vi "Curtin1.vi"() -> ()   [LabVIEW 2022 SP3]
uses:
  ViolinSubs/Curtin1_Label.ctl
  ViolinSubs/Mic/Mic_Global.vi
  ViolinSubs/GraphType.ctl
  ViolinSubs/Perspective/subs/Perspective_Globals.vi
  <vilib>/Utility/miscctls.llb/LVPoint32TypeDef.ctl
  <vilib>/Platform/browser.llb/Open URL in Default Browser (string).vi
panel:
  in  "microphone":bool
  in  "Device":u16(ring) items=["BuerginBase Microphone", "Onyx Producer 2-2", "MacBook Pro Microphone", "Camo Microphone", "KM Audio Device", "Microsoft Teams Audio", "ZoomAudioDevice"]
  out "comma?":bool
  out "startX":i32
  out "Ctrl":bool
  out "beta":string
  in  "Settings":u16(ring) items=["Settings...", "Preferences", "Templates", "Calibrations", "Live View", "Motor Cntrl"]
  in  "ScratchPads":u16(ring) items=["Scratch...", "accelerometer taptone Scratchpad", "Admittance Scratchpad", "Laser Admitance ScratchPad", "Radiation ScratchPad", "ScratchPad", "TapTones ScratchPad"]
  in  "New Test":u16(ring) items=["New Test...", "Admittance H", "Current Settings", "Internal mic H", "JC Admit H laser", "JC Admit.HV laser", "JC H 12 radiation", "JC H 7 radiation", "JC HV 24 radiation", "Radiation H 1", "Tap repeatabilty H20"]
  in  "Help":bool
  in  "About":bool
  in  "Start":bool
  in  "email":bool
  in  "Interpret":bool
  in  "Force YRescale":bool
  out "Complex Out":cluster{dbl, "df":dbl, cdb[]}[](array[cluster])
  out "# selected":i32
  in  "Fun":bool
  out "Version":string
  in  "Preferences":bool
  in  "Set Colors":bool
  in  "Colors":u16(ring) items=["Name Current...", "Last Saved", "24 Colors", "All black", "fered", "fred", "JC"]
  in  "Share":bool
  in  "Undo":bool
  in  "Clear All":bool
  in  "select all":bool
  in  "deselect":bool
  in  "Clear":bool
  in  "Lists":bool
  in  "Browse":bool
  in  "Search":bool
  in  "Redo":bool
  in  "Files":T1[](array[typedef])
  in  "zoom":bool
  in  "Mouse Down?":bool
  in  "Views":T3={"View Type"=0, "Smoothing"=0, "Bands"=0, "Edit"=FALSE, "rescale Y"=FALSE, "rescale X"=FALSE, "X_Low"=0.0, "X_High"=0.0, "dB Range"=40.0, "Excel"=FALSE, "Y Scaling"=TRUE, "X Scaling"=TRUE, "Plot"=0} {"Plot" items=["FRF", "rad phase unwrapped", "deg phase unwrapped", "rad phase wrapped", "deg phase wrapped", "White Plots", "MJ Map", "Real and Imaginary"]; "Bands" items=["No Bands", "1 Curtin 4 (200-780-1740-2930-7000)", "1 Curtin 4a (200-780-1740-2930-6000)", "1 Curtin 5  (200-780-1740-2930-7000-10000)", "1 Curtin 5b  (200-780-1740-2930-7000-20000)", "1 Curtin 5c (250-350-780-1740-2930-7000)", "1 Curtin 5c ()", "2 Curtin (200-7000)", "3 Curtin 10 (200-340-490-640-780-1150-1390-1730-2370-2930-7000)", "4 Curtin (200-780-7000)", "Bark  (200-300-400-510-630-770-920-1080-1270-1480-1720-2000-2320-2700-3150-3700-4400-5300-6400-7700-9500)", "Curtin 4a (250-780-1740-2930-7000)", "Dunnwald (190-650-1300-1640-2580-4200-6400)", "Dunnwald (190-650-1300-4200-6400)", "Gabriellson (200-650-1080-1270-2000-3000-3700-7000)", "ivci18 rad. efficiency (200-321-618-1841-2095-3484-7790)", "Meinel (280-650-2000-3000-7000)", "ObieAlto (200-650-1575-2450-6300)", "rad. efficiency ivci (200-345-730-1192-1875-2363-3033-4040-5673)"]; "Smoothing" items=["No smoothing"=0, "1/4 semitone"=25, "1/2 semitone"=50, "1 semitone"=100, "2 semitones"=200, "3 semitones"=300, "4 semitones"=400, "Octave"=1200, "Woodhouse"=19]; "View Type" items=["As measured"=0, "Normalize"=1, "Cplx Average"=3, "Real Average"=4, "Standard Deviation"=5]}
  out "Position":string
  in  "Color Table":T4(ring)=enum."Greyscale"
  out "MJPlot":dbl[][](graph)
  out "Coords":T5
  out "White Plots":picture
  out "FRF":cluster{"x0":dbl, "df":dbl, dbl[]}[](graph)
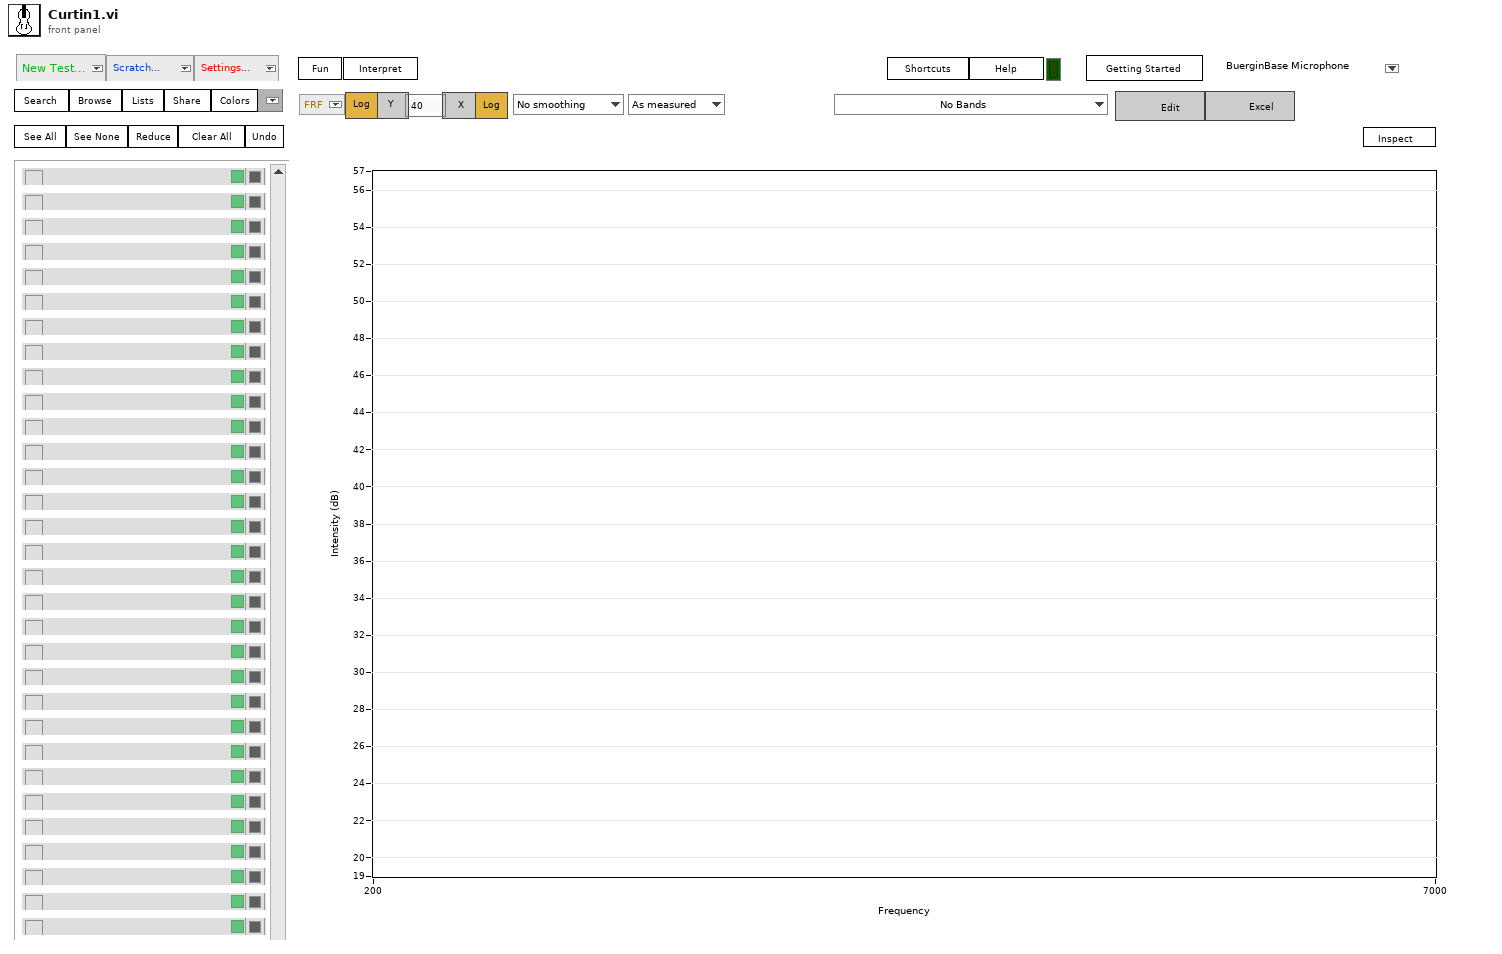
[diagram p1: front panel]
types:
  T1 = typedef "Curtin1_Label.ctl" = cluster{"Show?":bool, "Name":string, "Color":u32, "Path":path, "Show Notes":bool, "correlate":bool}
  T2 = typedef "GraphType.ctl" = u16
  T3 = cluster{"View Type":u16, "Smoothing":u16, "Bands":u16, "Edit":bool, "rescale Y":bool, "rescale X":bool, "X_Low":dbl, "X_High":dbl, "dB Range":dbl, "Excel":bool, "Y Scaling":bool, "X Scaling":bool, "Plot":T2}
  T4 = enum16{"Apricot", "Carnation", "Ether", "Greyscale", "Greyscale-banded", "Hot Metal", "Lava Waves", "Mac", "Morning Glory", "Rainbow", "Rainbow-banded", "Rainbow-inverted", "Rainbow-striped", "Saturn", "Seismic", "Space"}
  T5 = typedef "LVPoint32TypeDef.ctl" = cluster{"Horizontal":i32, "Vertical":i32}
  T6 = enum32{"SPL", "Voltage", "Accelerometer", "Vibrometer", "home", "Units"}
  T7 = enum16{"big-endian, network order", "native, host order", "little-endian"}
  T8 = enum16{"Grab Lines", "Grab Bands", "Grab Centroids"}
  T9 = cluster{"Alerts":bool, "Log X Axis":bool, "dB scale":bool, "Averaging":bool, "Fade":dbl, "Centroids?":bool, "line thickness":u8}
  T10 = typedef "LVBoundsTypeDef.ctl" = cluster{"Width":u32, "Height":u32}
  T11 = typedef "LVPositionTypeDef.ctl" = cluster{"Left":i32, "Top":i32}
  T12 = typedef "PreferencesControl.ctl" = cluster{"Name of test":string, "Date":timestamp, "Location":string, "Template":string, "Soundcard":string, "resolution":u16, "Sampling rate":u16, "Ch1 Gain ":dbl, "Ch2 Gain":dbl, "Sample time (s)":dbl, "Pre-trigger (s)":dbl, "Hammer Threshold":dbl, "Positions":i16, "Taps/Position":i16, "Set Names":string, "Freq resolution":dbl, "Hammer cutoff":dbl, "Mic cutoff":dbl, "Double bounce ":dbl, "Hammer Cal":dbl, "dB Offset":dbl, "Accel Cal":dbl, "Vibrometer Cal":dbl, "Mic Cal":dbl, "Output":u16, "Voltage Cal":dbl, "Vibrometer Port":refnum<visa-resource-name>, "Range":u16, "High Pass":u16, "Bandwidth":u16, "X Range":cluster{"Minimum":dbl, "Maximum":dbl, "Increment":dbl, "Minor Increment":dbl, "Start":dbl}[], "Y Range":cluster{"Minimum":dbl, "Maximum":dbl, "Increment":dbl, "Minor Increment":dbl, "Start":dbl}[], "dB Spread":dbl, "Trigger":u16, "Ch_1":u8, "Ch_2":u8, "flip?":bool, "60Hz":bool, "Time offset":dbl, "Piezo Cal":dbl, "Default Notes":string, "Tom":bool}
  T13 = typedef "eventvkey.ctl" = enum16{"ASCII", "Enter", "Return", "Shift", "Ctrl", "Alt", "Cmd", "Opt", "Caps", "NumLock", "Clear", "Break", "Up", "Down", "Left", "Right", "Insert", "Delete", "Home", "End", "PageUp", "PageDown", "Escape", "Help", "Pause", "ScrollLock", "F1", "F2", "F3", "F4", "F5", "F6", "F7", "F8", "F9", "F10", "F11", "F12", "F13", "F14", "F15", "F16", "F17", "F18", "F19", "F20", "F21", "F22", "F23", "F24", "Play", "VolumeUp", "VolumeDown", "Mute", "Two Byte Char"}
  T14 = typedef "LVMouseTypeDef.ctl" = cluster{"Mouse Position":cluster{"X":i32, "Y":i32}, "Mouse Modifiers":cluster{"Button Down":bool, "Shift Mod":bool, "Menu Mod":bool, "Option Mod":bool}}
  T15 = enum32{"Invalid", "Standard", "Closed", "Hidden", "Minimized", "Maximized"}
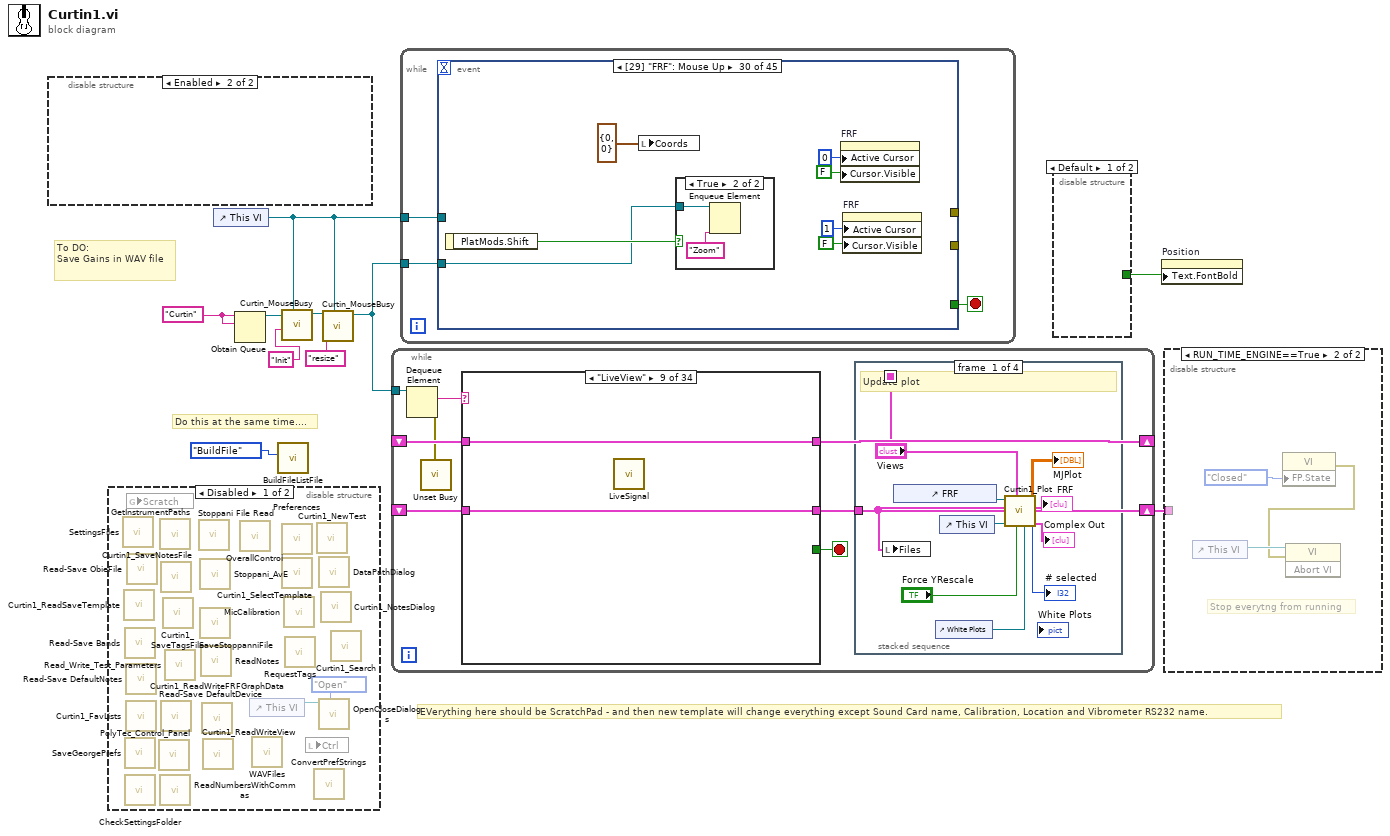
[diagram p0: block diagram]
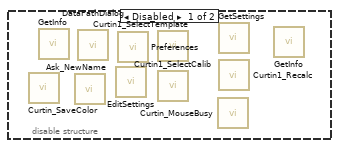
[diagram p2: hidden frame]
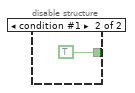
[diagram p4: hidden frame]
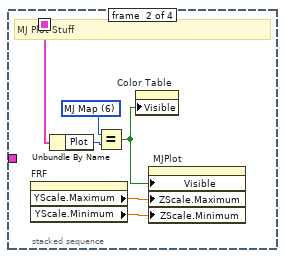
[diagram p6: hidden frame]
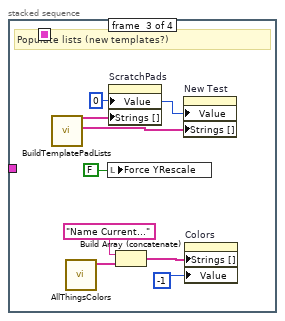
[diagram p7: hidden frame]
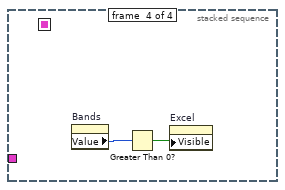
[diagram p8: hidden frame]
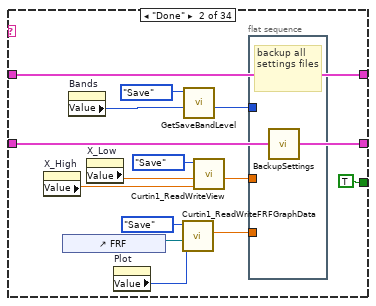
[diagram p10: hidden frame]
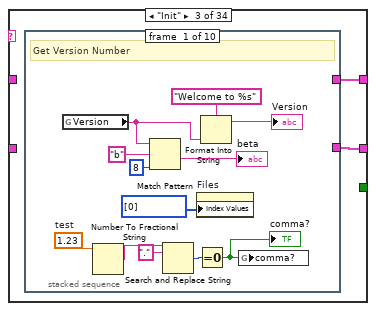
[diagram p11: hidden frame]
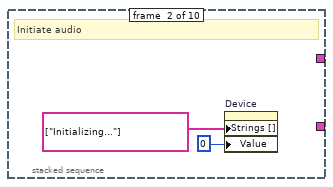
[diagram p12: hidden frame]
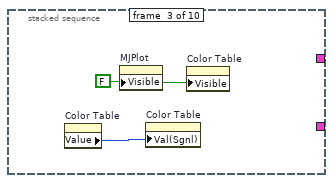
[diagram p13: hidden frame]
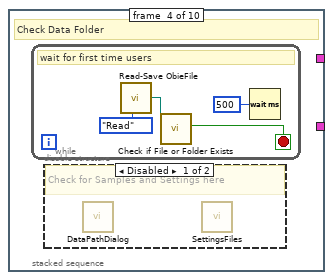
[diagram p14: hidden frame]
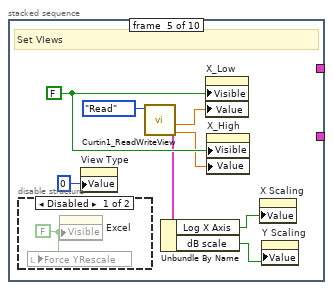
[diagram p16: hidden frame]
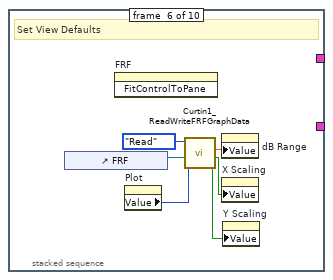
[diagram p18: hidden frame]
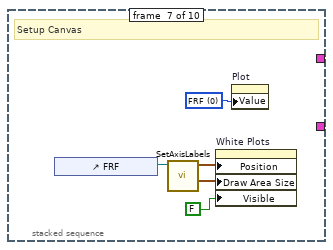
[diagram p19: hidden frame]
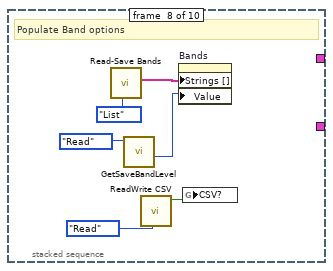
[diagram p20: hidden frame]
diagram:
  w8 = "Curtin" ("name (unnamed)")
  # "Do this at the same time...."
  # "To DO:\nSave Gains in WAV file"
  # "EVerything here should be ScratchPad - and then new template will change everything except Sound Card name, Calibration, Location and Vibrometer RS232 name."
  n1 = disable-structure shown="Enabled" {
    frame Disabled {
      n2 = call "Curtin_SaveColor.vi"() -> ()  [unwired: 10 in, 2 out]
      n3 = call "GetInfo.vi"() -> ()  [unwired: 11 in, 1 out]
      n4 = call "Ask_NewName.vi"() -> ()  [unwired: 10 in, 2 out]
      n5 = call "DataPathDialog.vi"() -> ()  [unwired: 10 in, 2 out]
      n6 = call "EditSettings.vi"() -> ()  [unwired: 10 in, 2 out]
      n7 = call "Preferences.vi"() -> ()  [unwired: 9 in, 3 out]
      n8 = call "Curtin1_SelectTemplate.vi"() -> ()  [unwired: 10 in, 2 out]
      n9 = call "Curtin1_SelectCalib.vi"() -> ()  [unwired: 11 in, 1 out]
      n10 = call "Curtin_MouseBusy.vi"() -> ()  [unwired: 11 in, 1 out]
      n11 = call "GetSettings.vi"() -> ()  [unwired: 10 in, 2 out]
      n12 = call "Curtin1_Recalc.vi"() -> ()  [unwired: 12 in]
      n13 = call "GetInfo.vi"() -> ()  [unwired: 11 in, 1 out]
    }
    frame Enabled {
    }
  }
  n14 = disable-structure shown="Disabled" {
    frame Disabled {
      n15 = call "SettingsFiles.vi"() -> ()  [unwired: 10 in, 2 out]
      n16 = call "Curtin1_ReadSaveTemplate.vi"() -> ()  [unwired: 8 in, 4 out]
      n17 = call "Read-Save Bands.vi"() -> ()  [unwired: 8 in, 4 out]
      n18 = call "SaveGeorgePrefs.vi"() -> ()  [unwired: 10 in, 2 out]
      n19 = call "CheckSettingsFolder.vi"() -> ()  [unwired: 12 in]
      n20 = call "Read-Save DefaultNotes.vi"() -> ()  [unwired: 10 in, 2 out]
      n21 = call "Curtin1_FavLists.vi"() -> ()  [unwired: 8 in, 4 out]
      n22 = global read "Mic_Global.vi" "Scratch"() -> ()  [unwired: 1 in]
      n23 = call "Read-Save ObieFile.vi"() -> ()  [unwired: 9 in, 3 out]
      n24 = call "PolyTec_Control_Panel.vi"() -> ()  [unwired: 9 in, 3 out]
      n25 = call "GetInstrumentPaths.vi"() -> ()  [unwired: 7 in, 5 out]
      n26 = call "ReadNumbersWithCommas.vi"() -> ()  [unwired: 8 in, 4 out]
      n27 = call "Curtin1_SaveNotesFile.vi"() -> ()  [unwired: 12 in]
      n28 = call "Read-Save DefaultDevice.vi"() -> ()  [unwired: 10 in, 2 out]
      n29 = call "Curtin1_SaveTagsFile.vi"() -> ()  [unwired: 12 in]
      n30 = call "Read_Write_Test_Parameters.vi"() -> ()  [unwired: 10 in, 2 out]
      n31 = call "Stoppani File Read.vi"() -> ()  [unwired: 3 in, 4 out]
      n32 = call "Stoppani_AvE.vi"() -> ()  [unwired: 8 in, 4 out]
      n33 = call "SaveStoppanniFile.vi"() -> ()  [unwired: 11 in, 1 out]
      n34 = call "ReadNotes.vi"() -> ()  [unwired: 10 in, 2 out]
      n35 = call "Curtin1_ReadWriteFRFGraphData.vi"() -> ()  [unwired: 9 in, 3 out]
      n36 = call "Curtin1_ReadWriteView.vi"() -> ()  [unwired: 9 in, 3 out]
      n37 = call "OverallControl.vi"() -> ()  [unwired: 10 in, 2 out]
      n38 = control-ref of="This VI"() -> (w11:refnum<vi>)
      n39 = call "WAVFiles.vi"() -> ()  [unwired: 8 in, 4 out]
      n40 = call "Preferences.vi"() -> ()  [unwired: 9 in, 3 out]
      n41 = call "Curtin1_SelectTemplate.vi"() -> ()  [unwired: 10 in, 2 out]
      n42 = call "MicCalibration.vi"() -> ()  [unwired: 11 in, 1 out]
      n43 = call "RequestTags.vi"() -> ()  [unwired: 11 in, 1 out]
      n44 = local read "Ctrl"() -> ()  [unwired: 1 in]
      n45 = call "ConvertPrefStrings.vi"() -> ()  [unwired: 10 in, 2 out]
      n46 = call "Curtin1_NewTest.vi"() -> ()  [unwired: 10 in, 2 out]
      n47 = call "DataPathDialog.vi"() -> ()  [unwired: 10 in, 2 out]
      n48 = call "OpenCloseDialogs.vi"("Task"=enum16{"Open", "Close"}."Open", "VI in"=w11) -> ()  [unwired: 8 in, 2 out]
      n49 = call "Curtin1_NotesDialog.vi"() -> ()  [unwired: 9 in, 3 out]
      n50 = call "Curtin1_Search.vi"() -> ()  [unwired: 10 in, 2 out]
    }
    frame Enabled {
    }
  }
  n51 = control-ref of="This VI"() -> (w3:refnum<vi>)
  n52 = Obtain Queue(name (unnamed)=w8, element data type=w8) -> (queue out=w7:refnum<queue>)  [unwired: 3 in, 2 out]
  n53 = call "BuildFileListFile.vi"("Task"=enum16{"BuildFile", "ReadFile"}."BuildFile") -> ()  [unwired: 9 in, 2 out]
  n54 = call "Curtin_MouseBusy.vi"("VI in"=w3, "element"="Init", "queue in"=w7) -> ("queue out"=w5:refnum<queue>)  [unwired: 8 in]
  n55 = call "Curtin_MouseBusy.vi"("VI in"=w3, "element"="resize", "queue in"=w5) -> ("queue out"=w6:refnum<queue>)  [unwired: 8 in]
  n56 = while {
    tunnel: w6 -> [w19]
    shift-right: [w16] -> w9
    shift-left: _ -> [w17]
    shift-right: [w14] -> _
    shift-left: _ -> [w15]
    stop <- w18 stop-if-true
    n57 = Dequeue Element(queue=w19) -> (element=w20:string, error out=w13:errorcluster)  [unwired: 2 in, 2 out]
    n58 = call <vilib>:"Unset Busy.vi"("error in (no error)"=w13) -> ()  [unwired: 10 in, 1 out]
    n59 = case shown="\"LiveView\"" w20 {
      selector: w20 -> [_ _ _ _ _ _ _ _ _ _ _ _ _ _ _ _ _ _ _ _ _ _ _ _ _ _ _ _ _ _ w301 w304 _ _]
      tunnel: [_ TRUE ("Discard?") _ _ _ _ _ _ _ _ _ _ _ _ _ _ _ _ _ _ _ _ _ _ _ _ _ _ _ _ _ _ _ _] -> w18
      tunnel: w17 -> [w48 w61 _ _ w129 w138 w154 w159 w161 w163 w165 w178 w185 w190 w201 w210 w222 w226 w228 w230 w234 w239 w242 w245 w258 w270 w276 w281 w286 w291 w302 w305 w312 w335]
      tunnel: [w48 w61 w63 w117 w129 w140 w154 w159 w161 w163 w169 w177 w186 w192 w196 w210 w221 w226 w228 w230 w232 w238 w241 w245 w257 w269 w275 w283 T1[] [] ("Files") w293 w302 w305 w312 w335] -> w16
      tunnel: [w47 w60 w64 w118 w132 w142 w155 w160 w162 w164 w167 w179 w187 w193 w202 w211 w224 w227 w229 w231 w235 w240 w243 w246 w259 w268 w274 w280 w287 w294 w303 w306 w316 w336] -> w14
      tunnel: w15 -> [w47 w60 _ w119 w132 w142 w155 w160 w162 w164 w168 w180 w188 w194 w203 w211 w225 w227 w229 w231 w236 w240 w243 w246 w260 w268 w274 w282 w289 w292 w303 w306 w316 w336]
      frame Default {
      }
      frame "Done" {
        n60 = property on="X_High" class="DigNum (strict)"() -> ("Value"=w55:dbl)  [unwired: 2 in, 2 out]
        n61 = control-ref of="FRF"() -> (w58:refnum<vi>)
        n62 = property on="Bands" class="Ring (strict)"() -> ("Value"=w53:u16)  [unwired: 2 in, 2 out]
        n63 = property on="X_Low" class="DigNum (strict)"() -> ("Value"=w56:dbl)  [unwired: 2 in, 2 out]
        n64 = property on="Plot" class="Ring (strict)"() -> ("Value"=w49:T2)  [unwired: 2 in, 2 out]
        n65 = call "Curtin1_ReadWriteFRFGraphData.vi"("Type"=w49, "FRF"=w58, "Task"=enum16{"Read", "Save"}."Save") -> ("dB"=w50:dbl)  [unwired: 6 in, 2 out]
        n66 = call "GetSaveBandLevel.vi"("Value in"=w53, "Task"=enum16{"Read", "Save"}."Save") -> ("Value out"=w52:u16)  [unwired: 9 in]
        n67 = call "Curtin1_ReadWriteView.vi"("X_High"=w55, "X_Low"=w56, "Task"=enum16{"Read", "Save"}."Save") -> ("X_Low out"=w51:dbl)  [unwired: 6 in, 2 out]
        n68 = flat-sequence {
          tunnel: w52 -> [_]
          tunnel: w51 -> [_]
          tunnel: w50 -> [_]
          frame #0 {
            # "backup all settings files"
            n69 = call "BackupSettings.vi"() -> ()  [unwired: 12 in]
          }
        }
      }
      frame "Init" {
        n70 = stacked-sequence {
          tunnel: [_ _ _ _ _ _ _ _ _ cluster{"files":T1[]}[] [] ("Array in")] -> w64
          tunnel: [_ _ _ _ _ _ _ _ _ T1[] [] ("Files")] -> w63
          frame #0 {
            w66 = 1.23  # test
            # "Get Version Number"
            n71 = global read "Mic_Global.vi" "Version"() -> (w70:string)
            n72 = Number To Fractional String(number=w66) -> (F-format string=w65:string)  [unwired: 3 in]
            n73 = Match Pattern(string=w70, regular expression="b", offset (0)=8) -> (after substring=→"beta":string)  [unwired: 3 out]
            n74 = Search and Replace String(input string=w65, search string=".") -> (number of replacements=w69:i32)  [unwired: 6 in, 3 out]
            n75 = property on="Files" class="Arr"("Index Values"=u32[] [0]) -> ()  [unwired: 2 in, 2 out]
            n76 = Equal To 0?(x=w69) -> (x = 0?=w67:bool)
            "comma?" <- w67
            n77 = Format Into String(format string="Welcome to %s", w70) -> (resulting string=→"Version":string)  [unwired: 2 in, 1 out]
            n78 = global write "Mic_Global.vi" "comma?"(w67) -> ()
          }
          frame #1 {
            # "Initiate audio"
            n79 = property on="Device" class="Ring (strict)"("Strings []"=string[] ["Initializing..."] ("Strings [4]"), "Value"=0) -> ()  [unwired: 2 in, 2 out]
          }
          frame #2 {
            w80 = FALSE ("Visible")
            n80 = property on="Color Table" class="Enum (strict)"() -> ("Value"=w79:T4)  [unwired: 2 in, 2 out]
            n81 = property on="MJPlot" class="IntGraph (strict)"("Visible"=w80) -> ()  [unwired: 2 in, 2 out]
            n82 = property on="Color Table" class="Enum (strict)"("Val(Sgnl)"=w79) -> ()  [unwired: 2 in, 2 out]
            n83 = property on="Color Table" class="Enum (strict)"("Visible"=w80) -> ()  [unwired: 2 in, 2 out]
          }
          frame #3 {
            # "Check Data Folder"
            n84 = while {
              stop <- w82 stop-if-true
              # "wait for first time users"
              n85 = call "Read-Save ObieFile.vi"("Task"=enum16{"Save", "Read"}."Read") -> ("DataPath Out"=w84:path)  [unwired: 8 in, 2 out]
              n86 = call <vilib>:"Check if File or Folder Exists.vi"("path"=w84) -> ("file or folder exists?"=w82:bool)  [unwired: 8 in, 2 out]
              n87 = Wait (ms)(milliseconds to wait=u32 500) -> ()  [unwired: 1 out]
            }
            n88 = disable-structure shown="Disabled" {
              frame Disabled {
                # "Check for Samples and Settings here"
                n89 = call "DataPathDialog.vi"() -> ()  [unwired: 10 in, 2 out]
                n90 = call "SettingsFiles.vi"() -> ()  [unwired: 10 in, 2 out]
              }
              frame Enabled {
              }
            }
          }
          frame #4 {
            w92 = FALSE ("Visible")
            # "Set VIews"
            n91 = disable-structure shown="Disabled" {
              frame Disabled {
                w93 = FALSE ("Visible")
                n92 = local write "Force YRescale"(w93) -> ()
                n93 = property on="Excel" class="Bool"("Visible"=w93) -> ()  [unwired: 2 in, 2 out]
              }
              frame Enabled {
              }
            }
            n94 = property on="View Type" class="Ring (strict)"("Value"=u16 0) -> ()  [unwired: 2 in, 2 out]
            n95 = call "Curtin1_ReadWriteView.vi"("Task"=enum16{"Read", "Save"}."Read") -> ("X_High out"=w89:dbl, "X_Low out"=w90:dbl, "View"=w85:T9)  [unwired: 8 in]
            n96 = Unbundle By Name(w85) -> ("Log X Axis"=w86:bool, "dB scale"=w87:bool)
            n97 = property on="X_Low" class="DigNum (strict)"("Visible"=w92, "Value"=w90) -> ()  [unwired: 2 in, 2 out]
            n98 = property on="X_High" class="DigNum (strict)"("Visible"=w92, "Value"=w89) -> ()  [unwired: 2 in, 2 out]
            n99 = property on="X Scaling" class="Bool (strict)"("Value"=w86) -> ()  [unwired: 2 in, 2 out]
            n100 = property on="Y Scaling" class="Bool (strict)"("Value"=w87) -> ()  [unwired: 2 in, 2 out]
          }
          frame #5 {
            # "Set View Defaults"
            n101 = control-ref of="FRF"() -> (w99:refnum<vi>)
            n102 = invoke on="FRF" class="WFGraph (strict)" method="FitControlToPane"() -> ()  [unwired: 3 in, 3 out]
            n103 = property on="Plot" class="Ring (strict)"() -> ("Value"=w96:T2)  [unwired: 2 in, 2 out]
            n104 = call "Curtin1_ReadWriteFRFGraphData.vi"("Type"=w96, "FRF"=w99, "Task"=enum16{"Read", "Save"}."Read") -> ("y log?"=w95:bool, "x log?"=w94:bool, "dB"=w97:dbl)  [unwired: 6 in]
            n105 = property on="dB Range" class="DigNum (strict)"("Value"=w97) -> ()  [unwired: 2 in, 2 out]
            n106 = property on="X Scaling" class="Bool (strict)"("Value"=w94) -> ()  [unwired: 2 in, 2 out]
            n107 = property on="Y Scaling" class="Bool (strict)"("Value"=w95) -> ()  [unwired: 2 in, 2 out]
          }
          frame #6 {
            w100 = T2 0 items=["FRF", "rad phase unwrapped", "deg phase unwrapped", "rad phase wrapped", "deg phase wrapped", "White Plots"] ("Value")
            # "Setup Canvas"
            n108 = control-ref of="FRF"() -> (w104:refnum<vi>)
            n109 = call "SetAxisLabels.vi"("WaveformGraph in"=w104) -> ("Bounds"=w102:T10, "Position"=w103:T11)  [unwired: 8 in, 1 out]
            n110 = property on="White Plots" class="Pict"("Position"=w103, "Draw Area Size"=w102, "Visible"=FALSE) -> ()  [unwired: 2 in, 2 out]
            n111 = property on="Plot" class="Ring (strict)"("Value"=w100) -> ()  [unwired: 2 in, 2 out]
          }
          frame #7 {
            # "Populate Band options"
            n112 = call "Read-Save Bands.vi"("Task"=enum16{"Save", "Read", "List"}."List") -> ("Long names"=w110:string[])  [unwired: 7 in, 3 out]
            n113 = call "GetSaveBandLevel.vi"("Task"=enum16{"Read", "Save"}."Read") -> ("Value out"=w107:u16)  [unwired: 10 in]
            n114 = call "ReadWrite CSV.vi"("Task"=enum16{"Save", "Read"}."Read") -> ("csv Out"=w105:bool)  [unwired: 10 in]
            n115 = property on="Bands" class="Ring (strict)"("Strings []"=w110, "Value"=w107) -> ()  [unwired: 2 in, 2 out]
            n116 = global write "Mic_Global.vi" "CSV?"(w105) -> ()
          }
          frame #8 {
            # "Always start everyone with ScratchPad \n\nRead the latest calibration but do not \ndo anything with it (no error code/saving)"
            # "Upload  ScratchPad template"
            n117 = call "UpdateScratchPad.vi"() -> ("Settings Out"=w112:T12)  [unwired: 10 in, 1 out]
            n118 = global write "Mic_Global.vi" "Settings"(w112) -> ()
            n119 = control-ref of="Device"() -> (w113:refnum<vi>)
            n120 = call "Curtin1_soundcards.vi"("hush?"=TRUE, "Settings In"=w112, "device:"=w113) -> ()  [unwired: 7 in, 2 out]
          }
          frame #9 {
            # "Initialize Undo and List"
          }
        }
      }
      frame "Update" {
        # "NOTE: info box is in this frame"
        n121 = call "Curtin1_NotesDialog.vi"("Files"="Files") -> ("Color"=w121:u32[], "removed?"=w120:bool, "Array"=w117:T1[])  [unwired: 8 in]
        n122 = call "Curtin1_Color.vi"("Color"=w121) -> ()  [unwired: 9 in, 2 out]
        n123 = case shown="True" w120 {
          tunnel: w119 -> [w123 w126]
          tunnel: [w123 w125] -> w118
          tunnel: w117 -> [_ w124]
          frame False {
          }
          frame True {
            # "removed a plot"
            n124 = call "Curtin_Undo.vi"("New Files"=w124, "Array in"=w126) -> ("Array out"=w125:cluster{"files":T1[]}[])  [unwired: 9 in]
          }
        }
        n125 = property on="Colors" class="Ring (strict)"("Value"=-1) -> ()  [unwired: 2 in, 2 out]
      }
      frame "Zoom" {
        n126 = for {
          tunnel: w129 -> [w135] mode=indexing
          tunnel: [w134] -> w128 mode=indexing if=w133
          n127 = Unbundle By Name(w135) -> ("Name"=w134:string, "Show?"=w133:bool)
        }
        n128 = property on="Plot" class="Ring (strict)"() -> ("Value"=w127:T2)  [unwired: 2 in, 2 out]
        n129 = property on="dB Range" class="DigNum (strict)"() -> ("Value"=w130:dbl)  [unwired: 2 in, 2 out]
        n130 = control-ref of="FRF"() -> (w131:refnum<vi>)
        n131 = call "GraphZoom.vi"("Plot"=w127, "Names"=w128, "dB Range"=w130, "Graph"=w131) -> ()  [unwired: 8 in]
      }
      frame "Preferences" {
        n132 = control-ref of="Files"() -> (w141:refnum<vi>)
        n133 = call "Preferences.vi"("FileList"=w141, "Files"=w138) -> ("Settings out"=w136:T12, "Success?"=w139:bool, "Fixed Files"=w137:T1[])  [unwired: 7 in]
        n134 = case shown="True" w139 {
          tunnel: w137 -> [_ w151]
          tunnel: [w143 w151] -> w140
          tunnel: w138 -> [w143 _]
          tunnel: w136 -> [_ w147]
          frame False {
          }
          frame True {
            n135 = global read "Mic_Global.vi" "View"() -> (w150:T9)
            n136 = call "UpdateScratchPad.vi"("Settings"=w147) -> ("Settings Out"=w144:T12)  [unwired: 9 in, 1 out]
            n137 = Unbundle By Name(w150) -> ("Log X Axis"=w149:bool, "dB scale"=w148:bool)
            n138 = control-ref of="Device"() -> (w146:refnum<vi>)
            n139 = call "Curtin1_soundcards.vi"("hush?"=TRUE, "Settings In"=w144, "device:"=w146) -> ()  [unwired: 7 in, 2 out]
            n140 = property on="X Scaling" class="Bool (strict)"("Value"=w149) -> ()  [unwired: 2 in, 2 out]
            n141 = property on="Y Scaling" class="Bool (strict)"("Value"=w148) -> ()  [unwired: 2 in, 2 out]
          }
        }
      }
      frame "Templates" {
        n142 = global read "Mic_Global.vi" "Scratch"() -> (w153:string)
        n143 = call "EditSettings.vi"("Template in"=w153) -> ("Settings out"=w152:T12)  [unwired: 9 in, 1 out]
        n144 = call "UpdateScratchPad.vi"("Settings"=w152) -> ()  [unwired: 9 in, 2 out]
      }
      frame "Calibrations" {
        # "Saves a new calib file\nand it is pushed in test"
        n145 = call "UpdateScratchPad.vi"() -> ("Settings Out"=w157:T12)  [unwired: 10 in, 1 out]
        n146 = call "MicCalibration.vi"("Type"=T6."home" ("Tyoe"), "Settings"=w157) -> ("Settings Out"=w156:T12)  [unwired: 9 in]
        n147 = global write "Mic_Global.vi" "Settings"(w156) -> ()
        n148 = call "UpdateScratchPad.vi"("Settings"=w156) -> ()  [unwired: 9 in, 2 out]
      }
      frame "LiveView" {
        n149 = call "LiveSignal.vi"() -> ()  [unwired: 12 in]
      }
      frame "MotorControl" {
        n150 = call "MotorControl.vi"() -> ()  [unwired: 12 in]
      }
      frame "Browse" {
        n151 = Array Size(array=w165) -> (size(s)=w166:i32)
        n152 = case shown="0" w166 {
          frame Default {
          }
          frame 0 {
            n153 = local write "Force YRescale"(TRUE ("Force YRescale")) -> ()
          }
        }
        n154 = call "Curtin_Undo.vi"("New Files"=w165, "Array in"=w168) -> ("Array out"=w167:cluster{"files":T1[]}[])  [unwired: 9 in]
        n155 = call "Curtin1_LoadFile.vi"("Files in"=w165) -> ("Files out"=w169:T1[])  [unwired: 10 in]
      }
      frame "Preload" {
        n156 = call "Curtin1_GlobalFolder.vi"() -> ("Samples"=w171:path)  [unwired: 1 in, 1 out]
        n157 = List Folder(path=w171, pattern="*.AvC") -> (path out=w174:path, filenames=w173:string[])  [unwired: 2 in, 2 out]
        n158 = call "Curtin_Undo.vi"("New Files"=w178, "Array in"=w180) -> ("Array out"=w179:cluster{"files":T1[]}[])  [unwired: 9 in]
        n159 = local write "Force YRescale"(TRUE ("Force YRescale")) -> ()
        n160 = for {
          tunnel: w174 -> [w183]
          tunnel: w173 -> [w182] mode=indexing
          tunnel: [w181] -> w172 mode=indexing
          n161 = Build Path(base path=w183, name or relative path=w182) -> (appended path=w181:path)
        }
        n162 = call "Curtin1_AddTest.vi"("Selected Paths"=w172) -> ("New Files"=w177:T1[])  [unwired: 10 in]
      }
      frame "Search" {
        n163 = Array Size(array=w185) -> (size(s)=w184:i32)
        n164 = case shown="0" w184 {
          frame Default {
          }
          frame 0 {
            n165 = local write "Force YRescale"(TRUE ("Force YRescale")) -> ()
          }
        }
        n166 = call "Curtin_Undo.vi"("New Files"=w185, "Array in"=w188) -> ("Array out"=w187:cluster{"files":T1[]}[])  [unwired: 9 in]
        n167 = call "Curtin1_Search.vi"("Old Files"=w185) -> ("New Files"=w186:T1[])  [unwired: 9 in, 1 out]
      }
      frame "Lists" {
        n168 = Array Size(array=w190) -> (size(s)=w191:i32)
        n169 = case shown="0" w191 {
          frame Default {
          }
          frame 0 {
            n170 = local write "Force YRescale"(TRUE ("Force YRescale")) -> ()
          }
        }
        n171 = call "Curtin_Undo.vi"("New Files"=w190, "Array in"=w194) -> ("Array out"=w193:cluster{"files":T1[]}[])  [unwired: 9 in]
        n172 = call "Curtin1_Lists.vi"("Old Files"=w190) -> ("New Files"=w192:T1[])  [unwired: 10 in]
      }
      frame "newColors" {
        n173 = property on="Colors" class="Ring (strict)"() -> ("Strings []"=w199:string[], "Value"=w200:u16)  [unwired: 2 in, 2 out]
        n174 = Index Array(array=w199, index=w200) -> (element=w198:string)
        n175 = call "AllThingsColors.vi"("Choice"=w198) -> ("Possible Colors"=w197:string[])  [unwired: 10 in]
        n176 = for {
          tunnel: w201 -> [w207] mode=indexing
          tunnel: [w206] -> w196 mode=indexing
          tunnel: w197 -> [_]
          i -> [w205]
          n177 = call "Curtin1_Color.vi"("Offset"=w205) -> ("New color"=w204:u32)  [unwired: 9 in, 1 out]
          n178 = Bundle By Name(cluster=w207, "Color"=w204) -> (w206:T1)
        }
        n179 = call "Curtin_Undo.vi"("New Files"=w201, "Array in"=w203) -> ("Array out"=w202:cluster{"files":T1[]}[])  [unwired: 9 in]
        n180 = local write "Files"(w196) -> ()
      }
      frame "saveColors" {
        n181 = call "Curtin_SaveColor.vi"() -> ("New Color"=w209:string, "Good?"=w208:bool)  [unwired: 10 in]
        n182 = case shown="True" w208 {
          tunnel: w210 -> [_ w215]
          tunnel: w209 -> [_ w213]
          tunnel: [_ w214] -> _
          frame False {
          }
          frame True {
            n183 = for {
              tunnel: w215 -> [w220] mode=indexing
              tunnel: [w219] -> w218 mode=indexing
              n184 = Unbundle By Name(w220) -> ("Color"=w219:u32)
            }
            n185 = call "GetColorFilePath.vi"("String"=w213) -> ("path"=w212:path)  [unwired: 9 in, 1 out]
            n186 = Write to Binary File(file (use dialog)=w212, data=w218, 5:FALSE ("prepend array or string size? (T)"), 9:T7."big-endian, network order" ("byte order (0:big-endian, network order)")) -> (error out=w214:errorcluster)  [unwired: 2 in, 2 out]
          }
        }
      }
      frame "setColors" {
        n187 = control-ref of="Files"() -> (w223:refnum<vi>)
        n188 = call "DefineColorPalette.vi"("Files in"=w222, "FileList"=w223) -> ("Files out"=w221:T1[])  [unwired: 9 in]
        n189 = call "Curtin_Undo.vi"("New Files"=w222, "Array in"=w225) -> ("Array out"=w224:cluster{"files":T1[]}[])  [unwired: 9 in]
      }
      frame "Fun" {
        n190 = call "FunArea.vi"("Old Files"=w226) -> ()  [unwired: 11 in]
      }
      frame "PlayIt" {
        n191 = call "PlayFile.vi"("Old Files"=w228) -> ()  [unwired: 11 in]
      }
      frame "Share" {
        n192 = call "Curtin1_Share.vi"("Files"=w230) -> ()  [unwired: 11 in]
      }
      frame "AppendTest" {
        n193 = global read "Mic_Global.vi" "Settings"() -> (w233:T12)
        n194 = call "Curtin1_DAQFiles.vi"("Settings"=w233, "Files in"=w234) -> ("Files out"=w232:T1[])  [unwired: 9 in]
        n195 = call "Curtin_Undo.vi"("New Files"=w234, "Array in"=w236) -> ("Array out"=w235:cluster{"files":T1[]}[])  [unwired: 9 in]
        n196 = flat-sequence {
          tunnel: w232 -> [_]
          frame #0 {
            n197 = call "BuildFileListFile.vi"("Task"=enum16{"BuildFile", "ReadFile"}."BuildFile") -> ()  [unwired: 9 in, 2 out]
          }
        }
      }
      frame "woodhouse" {
        n198 = call "Woodhouse.vi"("Files in"=w239) -> ("Files out"=w238:T1[])  [unwired: 10 in]
      }
      frame "SamZ" {
        n199 = call "SamZ_Format.vi"("Files in"=w242) -> ("Files out"=w241:T1[])  [unwired: 10 in]
      }
      frame "Folder" {
        n200 = for {
          tunnel: w245 -> [w251] mode=indexing
          tunnel: [w250] -> w244 mode=indexing if=w249
          n201 = Unbundle By Name(w251) -> ("Path"=w250:path, "Show?"=w249:bool)
        }
        n202 = for {
          tunnel: w244 -> [w248] mode=indexing
          n203 = Strip Path(path=w248) -> (stripped path=w247:path)  [unwired: 1 out]
          n204 = call "OpenFolder.vi"("LabVIEW Data Path"=w247) -> ()  [unwired: 11 in]
        }
      }
      frame "AppendAve" {
        n205 = local read "Complex Out"() -> (w256:cluster{dbl, "df":dbl, cdb[]}[])
        n206 = property on="View Type" class="Ring (strict)"() -> ("Value"=w254:u16)  [unwired: 2 in, 2 out]
        n207 = local read "# selected"() -> (w255:i32)
        n208 = call "SaveGroupAverages.vi"("nAverages"=w255, "Value"=w254, "Complex"=w256) -> ("New Path"=w252:path)  [unwired: 8 in]
        n209 = Not A Number/Path/Refnum?(number/path/refnum=w252) -> (NaN/Path/Refnum?=w253:bool)
        n210 = call "Curtin_Undo.vi"("New Files"=w258, "Array in"=w260) -> ("Array out"=w259:cluster{"files":T1[]}[])  [unwired: 9 in]
        n211 = case shown="False" w253 {
          tunnel: w258 -> [w265 w267]
          tunnel: [w264 w267] -> w257
          tunnel: w252 -> [w263 _]
          frame False {
            n212 = Build Array(w263) -> (w262:path[])
            n213 = call "Curtin1_AddTest.vi"("Old Files"=w265, "Selected Paths"=w262) -> ("New Files"=w264:T1[])  [unwired: 9 in]
            n214 = property on="View Type" class="Ring (strict)"("Val(Sgnl)"=0) -> ()  [unwired: 2 in, 2 out]
            n215 = call "BuildFileListFile.vi"("Task"=enum16{"BuildFile", "ReadFile"}."BuildFile") -> ()  [unwired: 9 in, 2 out]
          }
          frame True {
          }
        }
      }
      frame "Deselect" {
        n216 = for {
          tunnel: w270 -> [w273] mode=indexing
          tunnel: [w272] -> w269 mode=indexing
          n217 = Bundle By Name(cluster=w273, "Show?"=FALSE) -> (w272:T1)
        }
      }
      frame "SelectAll" {
        n218 = for {
          tunnel: w276 -> [w279] mode=indexing
          tunnel: [w278] -> w275 mode=indexing
          n219 = Bundle By Name(cluster=w279, "Show?"=TRUE) -> (w278:T1)
        }
      }
      frame "Clear" {
        n220 = call "Curtin_Undo.vi"("New Files"=w281, "Array in"=w282) -> ("Array out"=w280:cluster{"files":T1[]}[])  [unwired: 9 in]
        n221 = for {
          tunnel: w281 -> [w285] mode=indexing
          tunnel: [w285] -> w283 mode=indexing if=w284
          n222 = Unbundle By Name(w285) -> ("Show?"=w284:bool)
        }
      }
      frame "Clear All" {
        n223 = call "Curtin_Undo.vi"("New Files"=w286, "Array in"=w289) -> ("Array out"=w287:cluster{"files":T1[]}[])  [unwired: 9 in]
      }
      frame "Undo" {
        n224 = Array Size(array=w292) -> (size(s)=w290:i32)
        n225 = case shown="Default" w290 {
          tunnel: [w296 w300] -> w294
          tunnel: [w295 w297] -> w293
          tunnel: w292 -> [w296 w298]
          tunnel: w291 -> [w295 _]
          frame 0 {
          }
          frame Default {
            n226 = Delete From Array(array=w298) -> (deleted portion=w299:cluster{"files":T1[]}, array with subset deleted=w300:cluster{"files":T1[]}[])  [unwired: 2 in]
            n227 = Unbundle(w299) -> ("files"=w297:T1[])
          }
        }
      }
      frame "Left", "Right" {
        n228 = call "FadeLeftRight.vi"("Key"=w301) -> ()  [unwired: 11 in]
      }
      frame "Down", "Up" {
        n229 = call "ThicknessUpDown.vi"("Key"=w304) -> ()  [unwired: 11 in]
      }
      frame "BandEdit" {
        n230 = property on="Bands" class="Ring (strict)"() -> ("Strings []"=w314:string[], "Value"=w315:u16)  [unwired: 2 in, 2 out]
        n231 = for {
          tunnel: w312 -> [w321] mode=indexing
          tunnel: [w320] -> w311 mode=indexing if=w319
          n232 = Unbundle By Name(w321) -> ("Name"=w320:string, "Show?"=w319:bool)
        }
        n233 = Index Array(array=w314, index=w315) -> (element=w313:string)
        n234 = local read "FRF"() -> (w309:cluster{"x0":dbl, "df":dbl, dbl[]}[])
        n235 = Array Size(array=w311) -> (size(s)=w310:i32)
        n236 = call "ExtractBands.vi"("Task"=T8."Grab Lines", "lines"=w310, "plot in"=w309) -> ("plot out"=w308:cluster{dbl, "dt":dbl, "Y":dbl[]}[])  [unwired: 7 in, 1 out]
        n237 = call "BuildBandsList.vi"("Selected Band"=w313, "Average FRF"=w308) -> ("Name"=w318:string, "updated?"=w317:bool)  [unwired: 8 in]
        n238 = case shown="True" w317 {
          tunnel: w318 -> [_ w323]
          frame False {
          }
          frame True {
            n239 = call "Read-Save Bands.vi"("Task"=enum16{"Save", "Read", "List"}."List") -> ("Long names"=w324:string[])  [unwired: 7 in, 3 out]
            n240 = Search 1D Array(1D array=w324, element=w323) -> (index of element=w322:i32)  [unwired: 1 in]
            n241 = property on="Bands" class="Ring (strict)"("Strings []"=w324, "Value"=w322) -> ()  [unwired: 2 in, 2 out]
          }
        }
      }
      frame "resize" {
        n242 = property on="Show Notes" class="Bool"() -> ("Height"=w332:u32)  [unwired: 2 in, 2 out]
        n243 = property on="Pane 3" class="Pane"() -> ("Height"=w333:u32)  [unwired: 2 in, 2 out]
        n244 = control-ref of="FRF"() -> (w328:refnum<vi>)
        n245 = Add(x=u32 5, y=w332) -> (x+y=w331:u32)
        n246 = Divide(x=w333, y=w331) -> (x/y=w334:dbl)
        n247 = Round Toward -Infinity(1:w334) -> (0:w330:dbl)
        n248 = call "SetAxisLabels.vi"("WaveformGraph in"=w328) -> ("Bounds"=w326:T10, "Position"=w327:T11)  [unwired: 8 in, 1 out]
        n249 = property on="Files" class="Arr"("Number of Rows"=w330) -> ()  [unwired: 2 in, 2 out]
        n250 = property on="White Plots" class="Pict"("Position"=w327, "Draw Area Size"=w326) -> ()  [unwired: 2 in, 2 out]
      }
    }
    n251 = stacked-sequence {
      seq-local: ["Views" _ _ _] -> [_ w31 _ _]
      tunnel: w16 -> [w30 _ _ _]
      frame #0 {
        # "Update plot"
        n252 = local write "Files"(w30) -> ()
        n253 = control-ref of="FRF"() -> (w22:refnum<vi>)
        n254 = control-ref of="White Plots"() -> (w24:refnum<vi>)
        n255 = control-ref of="This VI"() -> (w28:refnum<vi>)
        n256 = call "Curtin1_Plot.vi"("Canvas 2"=w24, "Force YRescale"="Force YRescale", "Settings"="Views", "VI Refnum"=w28, "Files"=w30, "FRF"=w22) -> ("Complex Out"=→"Complex Out":cluster{dbl, "df":dbl, cdb[]}[], "size(s)"=→"# selected":i32, "Average FRF"=→"FRF":cluster{"x0":dbl, "df":dbl, dbl[]}[], "MJ Plot"=→"MJPlot":dbl[][])  [unwired: 2 in]
      }
      frame #1 {
        w35 = T2 6 items=["FRF", "rad phase unwrapped", "deg phase unwrapped", "rad phase wrapped", "deg phase wrapped", "White Plots", "MJ Map"] ("x")
        # "MJ Plot Stuff"
        n257 = property on="FRF" class="WFGraph (strict)"() -> ("YScale.Maximum"=w33:dbl, "YScale.Minimum"=w32:dbl)  [unwired: 2 in, 2 out]
        n258 = Unbundle By Name(w31) -> ("Plot"=w34:T2)
        n259 = Equal?(x=w35, y=w34) -> (x = y?=w36:bool)
        n260 = property on="Color Table" class="Enum (strict)"("Visible"=w36) -> ()  [unwired: 2 in, 2 out]
        n261 = property on="MJPlot" class="IntGraph (strict)"("Visible"=w36, "ZScale.Maximum"=w33, "ZScale.Minimum"=w32) -> ()  [unwired: 2 in, 2 out]
      }
      frame #2 {
        w38 = 0
        # "Populate lists (new templates?)"
        n262 = call "BuildTemplatePadLists.vi"() -> ("Templates"=w44:string[], "ScratchPads"=w39:string[])  [unwired: 8 in, 2 out]
        n263 = call "AllThingsColors.vi"() -> ("Possible Colors"=w42:string[])  [unwired: 11 in]
        n264 = local write "Force YRescale"(FALSE ("Force YRescale")) -> ()
        n265 = property on="ScratchPads" class="Ring (strict)"("Value"=w38, "Strings []"=w39) -> ()  [unwired: 2 in, 2 out]
        n266 = Build Array (concatenate)("Name Current...", w42) -> (w40:string[])
        n267 = property on="New Test" class="Ring (strict)"("Value"=w38, "Strings []"=w44) -> ()  [unwired: 2 in, 2 out]
        n268 = property on="Colors" class="Ring (strict)"("Strings []"=w40, "Value"=-1) -> ()  [unwired: 2 in, 2 out]
      }
      frame #3 {
        n269 = property on="Bands" class="Ring (strict)"() -> ("Value"=w46:u16)  [unwired: 2 in, 2 out]
        n270 = Greater Than 0?(x=w46) -> (x > 0?=w45:bool)
        n271 = property on="Excel" class="Bool"("Visible"=w45) -> ()  [unwired: 2 in, 2 out]
      }
    }
  }
  n272 = while {
    tunnel: w6 -> [w339]
    tunnel: w3 -> [w337]
    stop <- w338 stop-if-true
    n273 = event shown="[29] \"FRF\": Mouse Up" {
      selector: _ -> [_ _ _ _ _ _ _ _ _ _ _ _ _ _ _ _ _ _ _ _ _ _ _ _ _ _ _ _ _ _ _ _ _ _ _ _ _ _ _ _ _ _ _ _ _]
      dyn-events: _ -> [_ _ _ _ _ _ _ _ _ _ _ _ _ _ _ _ _ _ _ _ _ _ _ _ _ _ _ _ _ _ _ _ _ _ _ _ _ _ _ _ _ _ _ _ _]
      timeout: _ -> [_ _ _ _ _ _ _ _ _ _ _ _ _ _ _ _ _ _ _ _ _ _ _ _ _ _ _ _ _ _ _ _ _ _ _ _ _ _ _ _ _ _ _ _ _]
      tunnel: w339 -> [_ w340 w347 _ w362 w364 w367 w370 w374 w377 w380 w382 w386 w389 w392 w395 w398 w409 w424 _ w439 _ w457 _ w477 _ _ _ _ w509 _ _ w522 w546 _ w559 w564 w566 _ _ _ w576 w581 _ w588]
      tunnel: [_ w342 _ _ _ _ _ _ _ _ _ _ _ _ _ _ _ _ _ _ _ _ _ _ _ _ _ _ _ _ _ _ _ _ _ _ _ _ _ _ _ _ _ _ _] -> w338
      tunnel: w337 -> [_ w341 _ _ w361 w365 w366 w369 w372 w375 w378 w383 w385 w388 w390 w394 w396 w407 _ _ _ _ _ _ w476 _ _ _ _ _ _ _ w531 w545 _ w558 _ _ _ _ _ _ w582 _ _]
      tunnel: [_ _ _ _ _ _ _ _ _ _ _ _ _ _ _ _ _ _ _ _ _ _ _ _ _ _ _ _ _ _ _ _ _ _ _ _ _ _ _ _ _ _ _ w585 _] -> _
      tunnel: [_ _ _ _ _ _ _ _ _ _ _ _ _ _ _ _ _ _ _ w429 _ _ _ _ _ _ _ _ _ _ _ _ _ _ _ _ _ _ _ _ _ _ _ _ _] -> _
      event Timeout {
        n274 = event-data() -> ()  [unwired: 1 in, 3 out]
      }
      event Panel Close? {
        w342 = TRUE ("Discard?")
        n275 = event-data() -> ()  [unwired: 1 in, 4 out]
        n276 = call "Curtin_MouseBusy.vi"("VI in"=w341, "element"="Done", "queue in"=w340) -> ()  [unwired: 8 in, 1 out]
        n277 = event-data("Discard?"=w342) -> ()  [unwired: 1 in, 1 out]
      }
      event Key Down {
        n278 = event-data() -> ("VKey"=w348:T13, "PlatMods.Opt"=w346:bool, "PlatMods.Alt"=w345:bool)  [unwired: 1 in]
        n279 = Or(x=w346, y=w345) -> (x .or. y?=→"Ctrl":bool)
        n280 = case shown="\"Left\"" w348 {
          tunnel: w347 -> [_ w349 w351 w353 w355]
          frame Default {
          }
          frame "Left" {
            n281 = Enqueue Element(queue=w349, element="Left") -> ()  [unwired: 2 in, 3 out]
          }
          frame "Right" {
            n282 = Enqueue Element(queue=w351, element="Right") -> ()  [unwired: 2 in, 3 out]
          }
          frame "Up" {
            n283 = Enqueue Element(queue=w353, element="Up") -> ()  [unwired: 2 in, 3 out]
          }
          frame "Down" {
            n284 = Enqueue Element(queue=w355, element="Down") -> ()  [unwired: 2 in, 3 out]
          }
        }
      }
      event Key Up {
        n285 = event-data() -> ("PlatMods.Alt"=w359:bool, "PlatMods.Opt"=w358:bool)  [unwired: 1 in]
        n286 = Or(x=w359, y=w358) -> (x .or. y?=w357:bool)
        n287 = local write "Ctrl"(w357) -> ()
      }
      event Panel Resize {
        n288 = event-data() -> ()  [unwired: 1 in, 1 out]
        n289 = call "Curtin_MouseBusy.vi"("VI in"=w361, "element"="resize", "queue in"=w362) -> ()  [unwired: 8 in, 1 out]
      }
      event "Browse": Value Change {
        n290 = event-data() -> ()  [unwired: 1 in, 1 out]
        n291 = call "Curtin_MouseBusy.vi"("VI in"=w365, "element"="Browse", "queue in"=w364) -> ()  [unwired: 8 in, 1 out]
      }
      event "Search": Value Change {
        n292 = event-data() -> ()  [unwired: 1 in, 1 out]
        n293 = call "Curtin_MouseBusy.vi"("VI in"=w366, "element"="Search", "queue in"=w367) -> ()  [unwired: 8 in, 1 out]
      }
      event "deselect": Value Change {
        n294 = event-data() -> ()  [unwired: 1 in, 1 out]
        n295 = call "Curtin_MouseBusy.vi"("VI in"=w369, "element"="Deselect", "queue in"=w370) -> ()  [unwired: 8 in, 1 out]
      }
      event "select all": Value Change {
        n296 = event-data() -> ()  [unwired: 1 in, 1 out]
        n297 = call "Curtin_MouseBusy.vi"("VI in"=w372, "element"="SelectAll", "queue in"=w374) -> ()  [unwired: 8 in, 1 out]
      }
      event "Undo": Value Change {
        n298 = event-data() -> ()  [unwired: 1 in, 1 out]
        n299 = call "Curtin_MouseBusy.vi"("VI in"=w375, "element"="Undo", "queue in"=w377) -> ()  [unwired: 8 in, 1 out]
      }
      event "Redo": Value Change {
        n300 = event-data() -> ()  [unwired: 1 in, 1 out]
        n301 = call "Curtin_MouseBusy.vi"("VI in"=w378, "element"="Redo", "queue in"=w380) -> ()  [unwired: 8 in, 1 out]
      }
      event "Clear": Value Change {
        n302 = event-data() -> ()  [unwired: 1 in, 1 out]
        n303 = call "Curtin_MouseBusy.vi"("VI in"=w383, "element"="Clear", "queue in"=w382) -> ()  [unwired: 8 in, 1 out]
      }
      event "Files": Value Change {
        n304 = event-data() -> ()  [unwired: 1 in, 1 out]
        n305 = call "Curtin_MouseBusy.vi"("VI in"=w385, "element"="Update", "queue in"=w386) -> ()  [unwired: 8 in, 1 out]
      }
      event "Clear All": Value Change {
        n306 = event-data() -> ()  [unwired: 1 in, 3 out]
        n307 = call "Curtin_MouseBusy.vi"("VI in"=w388, "element"="Clear All", "queue in"=w389) -> ()  [unwired: 8 in, 1 out]
      }
      event "Lists": Value Change {
        n308 = event-data() -> ()  [unwired: 1 in, 1 out]
        n309 = call "Curtin_MouseBusy.vi"("VI in"=w390, "element"="Lists", "queue in"=w392) -> ()  [unwired: 8 in, 1 out]
      }
      event "Share": Value Change {
        n310 = event-data() -> ()  [unwired: 1 in, 1 out]
        n311 = call "Curtin_MouseBusy.vi"("VI in"=w394, "element"="Share", "queue in"=w395) -> ()  [unwired: 8 in, 1 out]
      }
      event "Colors": Value Change {
        n312 = event-data() -> ()  [unwired: 1 in, 2 out]
        n313 = case shown="0" "Colors" {
          tunnel: w398 -> [w401 w406]
          tunnel: w396 -> [w399 w402]
          frame 0 {
            n314 = call "Curtin_MouseBusy.vi"("VI in"=w399, "element"="saveColors", "queue in"=w401) -> ()  [unwired: 8 in, 1 out]
          }
          frame Default {
            n315 = call "Curtin_MouseBusy.vi"("VI in"=w402, "element"="newColors", "queue in"=w406) -> ("queue out"=w404:refnum<queue>)  [unwired: 8 in]
            n316 = call "Curtin_MouseBusy.vi"("VI in"=w402, "element"="Update", "queue in"=w404) -> ()  [unwired: 8 in, 1 out]
          }
        }
      }
      event "Set Colors": Value Change {
        n317 = event-data() -> ()  [unwired: 1 in, 1 out]
        n318 = call "Curtin_MouseBusy.vi"("VI in"=w407, "element"="setColors", "queue in"=w409) -> ()  [unwired: 8 in, 1 out]
        n319 = disable-structure shown="Disabled" {
          disable-tunnel: _ -> [w410 _]
          frame Disabled {
            n320 = Enqueue Element(queue=w410, element="Update") -> ()  [unwired: 2 in, 3 out]
          }
          frame Enabled {
          }
        }
      }
      event "Views": Value Change {
        n321 = event-data() -> ("NewVal"=w412:T3)  [unwired: 1 in]
        n322 = Unbundle By Name(w412) -> ("X Scaling"=w419:bool, "Y Scaling"=w418:bool, "View Type"=w423:u16, "Edit"=w414:bool)
        n323 = global read "Mic_Global.vi" "View"() -> (w420:T9)
        n324 = Bundle By Name(cluster=w420, "Log X Axis"=w419, "dB scale"=w418) -> (w417:T9)
        n325 = Select(t="BandEdit" ("element"), s=w414, f="Update" ("element")) -> (s? t:f=w413:string)
        n326 = Enqueue Element(queue=w424, element=w413) -> ()  [unwired: 2 in, 3 out]
        n327 = global write "Mic_Global.vi" "View"(w417) -> ()
        n328 = Equal?(x=u16 1 ("View Type"), y=w423) -> (x = y?=w421:bool)
        n329 = property on="X_Low" class="DigNum (strict)"("Visible"=w421) -> ()  [unwired: 2 in, 2 out]
        n330 = property on="X_High" class="DigNum (strict)"("Visible"=w421) -> ()  [unwired: 2 in, 2 out]
      }
      event "Views.dB Range": Value Change {
        n331 = event-data() -> ()  [unwired: 1 in, 1 out]
        n332 = control-ref of="FRF"() -> (w428:refnum<vi>)
        n333 = property class="WFGraph (strict)"(reference=w428) -> (reference out=w431:refnum<vi>, error out=w430:errorcluster, "YScale.Maximum"=w434:dbl)  [unwired: 1 in]
        n334 = property on="dB Range" class="DigNum (strict)"() -> ("Value"=w433:dbl)  [unwired: 2 in, 2 out]
        n335 = Subtract(x=w434, y=w433) -> (x-y=w432:dbl)
        n336 = property class="WFGraph (strict)"(reference=w431, error in=w430, "YScale.Minimum"=w432) -> (reference out=w427:refnum<vi>, error out=w429:errorcluster)
        n337 = property on="Plot" class="Ring (strict)"() -> ("Value"=w426:T2)  [unwired: 2 in, 2 out]
        n338 = call "Curtin1_ReadWriteFRFGraphData.vi"("Type"=w426, "FRF"=w427, "Task"=enum16{"Read", "Save"}."Save") -> ()  [unwired: 6 in, 3 out]
      }
      event "Views.View Type": Value Change {
        n339 = event-data() -> ("NewVal"=w436:u16)  [unwired: 1 in]
        n340 = disable-structure shown="Disabled" {
          disable-tunnel: w439 -> [w440 _]
          frame Disabled {
            n341 = Enqueue Element(queue=w440, element="Update") -> ()  [unwired: 2 in, 3 out]
          }
          frame Enabled {
          }
        }
        n342 = Equal?(x=u16 1 ("View Type"), y=w436) -> (x = y?=w438:bool)
        n343 = property on="X_Low" class="DigNum (strict)"("Visible"=w438) -> ()  [unwired: 2 in, 2 out]
        n344 = property on="X_High" class="DigNum (strict)"("Visible"=w438) -> ()  [unwired: 2 in, 2 out]
        n345 = local write "Force YRescale"(TRUE ("Force YRescale")) -> ()
      }
      event Value Change {
        n346 = event-data() -> ("NewVal"=w442:T2, "OldVal"=w443:T2)  [unwired: 1 in]
        n347 = stacked-sequence {
          tunnel: w443 -> [w444 _]
          tunnel: w442 -> [_ w448]
          frame #0 {
            n348 = control-ref of="FRF"() -> (w446:refnum<vi>)
            n349 = call "Curtin1_ReadWriteFRFGraphData.vi"("Type"=w444, "FRF"=w446, "Task"=enum16{"Read", "Save"}."Save") -> ()  [unwired: 6 in, 3 out]
          }
          frame #1 {
            w449 = T2 5 items=["FRF", "rad phase unwrapped", "deg phase unwrapped", "rad phase wrapped", "deg phase wrapped", "White Plots"] ("y")
            # "There is a bug in LV so runs twice\none for changing Views and again\nfor changing scaling value..."
            n350 = control-ref of="FRF"() -> (w452:refnum<vi>)
            n351 = Equal?(x=w448, y=w449) -> (x = y?=w450:bool)
            n352 = call "Curtin1_ReadWriteFRFGraphData.vi"("Type"=w448, "FRF"=w452, "Task"=enum16{"Read", "Save"}."Read") -> ("y log?"=w455:bool, "x log?"=w454:bool, "dB"=w453:dbl)  [unwired: 6 in]
            n353 = property on="White Plots" class="Pict"("Visible"=w450) -> ()  [unwired: 2 in, 2 out]
            n354 = property on="dB Range" class="DigNum (strict)"("Value"=w453) -> ()  [unwired: 2 in, 2 out]
            n355 = property on="X Scaling" class="Bool (strict)"("Value"=w454) -> ()  [unwired: 2 in, 2 out]
            n356 = local write "Force YRescale"(TRUE ("Force YRescale")) -> ()
            n357 = property on="Y Scaling" class="Bool (strict)"("Val(Sgnl)"=w455) -> ()  [unwired: 2 in, 2 out]
          }
        }
      }
      event "White Plots": Mouse Move {
        n358 = event-data() -> ()  [unwired: 1 in, 1 out]
        n359 = property on="White Plots" class="Pict"() -> ("Width"=w458:u32, "Mouse"=w460:T14)  [unwired: 2 in, 2 out]
        n360 = Unbundle By Name(w460) -> ("Mouse Position.X"=w456:i32, "Mouse Modifiers.Button Down"=w459:bool)
        n361 = case shown="True" w459 {
          tunnel: w456 -> [_ w471]
          tunnel: w458 -> [_ w470]
          tunnel: w457 -> [_ w468]
          tunnel: w456 -> [_ w467]
          frame False {
          }
          frame True {
            n362 = local read "startX"() -> (w466:i32)
            n363 = Divide(x=w471, y=w470) -> ()  [unwired: 1 out]
            n364 = Subtract(x=w467, y=w466) -> (x-y=w465:i32)
            n365 = Enqueue Element(queue=w468, element="Update") -> ()  [unwired: 2 in, 3 out]
            n366 = Bundle(w465, "y"=0) -> (w462:cluster{i32, "y":i32})  [unwired: 1 in]
            n367 = Add(x=cluster{"x":dbl, "y":dbl}[] [{"x"=-400.0, "y"=200.0}, {"x"=400.0, "y"=200.0}] ("vanishing points"), y=w462) -> (x+y=w461:cluster{dbl, "y":dbl}[])
            n368 = global write "Perspective_Globals.vi" "vanishing points"(w461) -> ()
          }
        }
      }
      event "White Plots": Mouse Down; "White Plots": Mouse Enter {
        n369 = event-data() -> ()  [unwired: 1 in, 4 out]
        n370 = property on="White Plots" class="Pict" props=["Width", "Mouse"]() -> ("Mouse"=w474:T14)  [unwired: 2 in, 3 out]
        n371 = Unbundle By Name(w474) -> ("Mouse Position.X"=→"startX":i32, "Mouse Modifiers.Button Down"=w473:bool)
        n372 = global write "Perspective_Globals.vi" "Outlines?"(w473) -> ()
      }
      event "White Plots": Mouse Leave; "White Plots": Mouse Up {
        n373 = event-data() -> ()  [unwired: 1 in, 1 out]
        n374 = call "Curtin_MouseBusy.vi"("VI in"=w476, "element"="Update", "queue in"=w477) -> ()  [unwired: 8 in, 1 out]
        n375 = global write "Perspective_Globals.vi" "Outlines?"(FALSE ("Outlines?")) -> ()
      }
      event "Color Table": Value Change {
        n376 = event-data() -> ()  [unwired: 1 in, 6 out]
        n377 = call "ColorTables.vi"("Color Table"="Color Table") -> ("Color Table Out"=w482:u32[])  [unwired: 2 in]
        n378 = property on="MJPlot" class="IntGraph (strict)"("Color Table"=w482, "ZScale.Low Color"=u32 16777215 ("Z Scale.Low Color"), "ZScale.Interpolate Color"=TRUE ("Z Scale.Interpolate Color"), "ZScale.High Color"=u32 0 ("Z Scale.High Color")) -> ()  [unwired: 2 in, 2 out]
      }
      event "FRF": Mouse Move {
        n379 = event-data() -> ("CtlRef"=w489:refnum<vi>, "Coords"=w488:T5)  [unwired: 1 in]
        n380 = local read "Coords"() -> (w484:T5)
        n381 = property on="Plot" class="Ring (strict)"() -> ("Value"=w485:T2)  [unwired: 2 in, 2 out]
        n382 = case shown="True" "Mouse Down?" {
          tunnel: w489 -> [_ w496]
          tunnel: w488 -> [_ w492]
          tunnel: ["" ("Position") w495] -> w487
          tunnel: w485 -> [_ w493]
          tunnel: w484 -> [_ w491]
          frame False {
          }
          frame True {
            n383 = local read "Ctrl"() -> (w494:bool)
            n384 = call "Cursor Values.vi"("Plot"=w493, "option?"=w494, "Start Coord"=w491, "Coords"=w492, "WaveformGraph in"=w496) -> ("Position"=w495:string)  [unwired: 6 in]
          }
        }
        "Position" <- w487
      }
      event "FRF": Mouse Enter {
        n385 = event-data() -> ()  [unwired: 1 in, 1 out]
        n386 = local write "Mouse Down?"(TRUE ("Mouse Down?")) -> ()
      }
      event "FRF": Mouse Leave {
        n387 = event-data() -> ()  [unwired: 1 in, 1 out]
        n388 = local write "Mouse Down?"(FALSE ("Mouse Down?")) -> ()
        n389 = local write "Coords"(T5 {"Horizontal"=0, "Vertical"=0} ("Coords")) -> ()
        n390 = property on="FRF" class="WFGraph (strict)"("Active Cursor"=u32 0, "Cursor.Visible"=FALSE) -> ()  [unwired: 2 in, 2 out]
        n391 = property on="FRF" class="WFGraph (strict)"("Active Cursor"=u32 1, "Cursor.Visible"=FALSE) -> ()  [unwired: 2 in, 2 out]
      }
      event "FRF": Mouse Up {
        n392 = event-data() -> ("PlatMods.Shift"=w510:bool)  [unwired: 1 in]
        n393 = local write "Coords"(T5 {"Horizontal"=0, "Vertical"=0} ("Coords")) -> ()
        n394 = case shown="True" w510 {
          tunnel: w509 -> [_ w511]
          frame False {
          }
          frame True {
            n395 = Enqueue Element(queue=w511, element="Zoom") -> ()  [unwired: 2 in, 3 out]
          }
        }
        n396 = property on="FRF" class="WFGraph (strict)"("Active Cursor"=u32 0, "Cursor.Visible"=FALSE) -> ()  [unwired: 2 in, 2 out]
        n397 = property on="FRF" class="WFGraph (strict)"("Active Cursor"=u32 1, "Cursor.Visible"=FALSE) -> ()  [unwired: 2 in, 2 out]
      }
      event "FRF": Mouse Down {
        n398 = event-data() -> ("PlatMods.Ctrl"=w515:bool, "Coords"=→"Coords":T5)  [unwired: 1 in]
        n399 = Not(x=w515) -> (.not. x?=w513:bool)
        n400 = disable-structure shown="Disabled" {
          disable-tunnel: w513 -> [w516 _]
          frame Disabled {
            n401 = property on="FRF" class="WFGraph (strict)"("Active Cursor"=u32 0, "Cursor.Visible"=w516) -> ()  [unwired: 2 in, 2 out]
            n402 = property on="FRF" class="WFGraph (strict)"("Active Cursor"=u32 1, "Cursor.Visible"=w516) -> ()  [unwired: 2 in, 2 out]
          }
          frame Enabled {
          }
        }
      }
      event "FRF": Scale Range Change {
        n403 = event-data() -> ("CtlRef"=w520:refnum<vi>)  [unwired: 1 in]
        n404 = property on="Plot" class="Ring (strict)"() -> ("Value"=w519:T2)  [unwired: 2 in, 2 out]
        n405 = call "Curtin1_ReadWriteFRFGraphData.vi"("Type"=w519, "FRF"=w520, "Task"=enum16{"Read", "Save"}."Save") -> ()  [unwired: 6 in, 3 out]
      }
      event "New Test", "ScratchPads": Value Change {
        n406 = event-data() -> ()  [unwired: 1 in, 1 out]
        n407 = property on="ScratchPads" class="Ring (strict)"() -> ("Strings []"=w530:string[])  [unwired: 2 in, 2 out]
        n408 = property on="New Test" class="Ring (strict)"() -> ("Strings []"=w529:string[])  [unwired: 2 in, 2 out]
        n409 = Index Array(array=w530, index="ScratchPads") -> (element=w526:string)
        n410 = Index Array(array=w529, index="New Test") -> (element=w527:string)
        n411 = case shown="Default" "ScratchPads" {
          tunnel: w522 -> [_ w535]
          frame 0 {
            # "New Test"
          }
          frame Default {
            # "Clear old"
            n412 = Enqueue Element(queue=w535, element="Clear All") -> ()  [unwired: 2 in, 3 out]
          }
        }
        n413 = Not Equal To 0?(x="New Test") -> (x != 0?=w528:bool)
        n414 = Select(t=w527, s=w528, f=w526) -> (s? t:f=w525:string)
        n415 = flat-sequence {
          tunnel: w525 -> [_]
          frame #0 {
            w536 = 0
            n416 = local write "ScratchPads"(w536) -> ()
            n417 = local write "New Test"(w536) -> ()
          }
        }
        n418 = call "ScratchOrNew.vi"("Template"=w525) -> ("Success"=w533:bool, "Settings Out"=w532:T12)  [unwired: 9 in]
        n419 = case shown="True" w533 {
          tunnel: w532 -> [_ w540]
          tunnel: w522 -> [_ w539]
          tunnel: w531 -> [_ w538]
          frame False {
          }
          frame True {
            n420 = call "Curtin1_Acquire.vi"("MainVI"=w538, "Settings"=w540) -> ("Data?"=w537:bool)  [unwired: 7 in, 2 out]
            n421 = case shown="True" w537 {
              tunnel: w539 -> [_ w542]
              frame False {
                # "No data taken"
                n422 = call "Ask_delete.vi"() -> ()  [unwired: 12 in]
              }
              frame True {
                # "success"
                n423 = Enqueue Element(queue=w542, element="AppendTest") -> ()  [unwired: 2 in, 3 out]
              }
            }
          }
        }
      }
      event "Start": Value Change {
        n424 = event-data() -> ()  [unwired: 1 in, 1 out]
        n425 = call "Startup Wizard.vi"() -> ("analysis?"=w543:string, "Settings"=w544:T12)  [unwired: 10 in]
        n426 = case shown="\"acq\"" w543 {
          tunnel: w546 -> [w550 w554 _]
          tunnel: w545 -> [w549 _ _]
          tunnel: w544 -> [w548 _ _]
          frame "acq" {
            n427 = call "Curtin1_Acquire.vi"("MainVI"=w549, "Settings"=w548) -> ("Data?"=w547:bool)  [unwired: 7 in, 2 out]
            n428 = case shown="True" w547 {
              tunnel: w550 -> [_ w552]
              frame False {
                # "No data taken"
                n429 = call "Ask_delete.vi"() -> ()  [unwired: 12 in]
              }
              frame True {
                n430 = Enqueue Element(queue=w552, element="AppendTest") -> ()  [unwired: 2 in, 3 out]
              }
            }
          }
          frame "analysis" {
            n431 = Enqueue Element(queue=w554, element="Preload") -> ()  [unwired: 2 in, 3 out]
          }
          frame Default {
          }
        }
      }
      event "Help": Value Change {
        n432 = event-data() -> ()  [unwired: 1 in, 1 out]
        n433 = fn#1354() -> (1:w556:bool)  [unwired: 1 out]
        n434 = Not(x=w556) -> (.not. x?=w555:bool)
        n435 = Control Help Window(1:w555) -> ()  [unwired: 1 in]
      }
      event "Preferences": Value Change {
        n436 = event-data() -> ()  [unwired: 1 in, 1 out]
        n437 = call "Curtin_MouseBusy.vi"("VI in"=w558, "element"="Preferences", "queue in"=w559) -> ()  [unwired: 8 in, 1 out]
      }
      event "Settings": Value Change {
        w560 = u16 0 items=["Settings...", "Preferences", "Templates", "Calibrations"] ("Settings")
        n438 = event-data() -> ()  [unwired: 1 in, 1 out]
        n439 = Index Array(array=string[] ["", "Preferences", "Templates", "Calibrations", "LiveView", "MotorControl"], index="Settings") -> (element=w561:string)
        n440 = Enqueue Element(queue=w564, element=w561) -> ()  [unwired: 2 in, 3 out]
        n441 = local write "Settings"(w560) -> ()
      }
      event "zoom": Value Change {
        n442 = event-data() -> ()  [unwired: 1 in, 1 out]
        n443 = Enqueue Element(queue=w566, element="Zoom") -> ()  [unwired: 2 in, 3 out]
      }
      event "email": Value Change {
        n444 = event-data() -> ()  [unwired: 1 in, 1 out]
        n445 = call-poly <vilib>:"Open URL in Default Browser.vi"("URL"="https://sites.google.com/view/oberlinacoustics/contactbug-reports") -> ()  [unwired: 5 in, 2 out]
      }
      event "About": Value Change {
        n446 = event-data() -> ()  [unwired: 1 in, 1 out]
        n447 = call "ObieHelp.vi"() -> ()  [unwired: 12 in]
      }
      event "Interpret": Value Change {
        n448 = event-data() -> ()  [unwired: 1 in, 1 out]
        n449 = property on="Bands" class="Ring (strict)"() -> ("Value"=w570:u16)  [unwired: 2 in, 2 out]
        n450 = local read "FRF"() -> (w568:cluster{"x0":dbl, "df":dbl, dbl[]}[])
        n451 = case shown="Default" w570 {
          tunnel: [w571 w572] -> w569
          tunnel: w568 -> [w571 w574]
          frame 0 {
          }
          frame Default {
            n452 = Array Size(array=w574) -> (size(s)=w575:i32)
            n453 = expression code="x*2/3"(w575) -> (w573:i32)
            n454 = Split 1D Array(array=w574, index=w573) -> (second subarray=w572:cluster{"x0":dbl, "df":dbl, dbl[]}[])  [unwired: 1 out]
          }
        }
        n455 = call "Explainations.vi"("FRF"=w569) -> ()  [unwired: 11 in]
      }
      event "Fun": Value Change {
        n456 = event-data() -> ()  [unwired: 1 in, 1 out]
        n457 = Enqueue Element(queue=w576, element="Fun") -> ()  [unwired: 2 in, 3 out]
      }
      event "microphone": Value Change {
        (unwired) "Preferences" ("element")
        n458 = event-data() -> ()  [unwired: 1 in, 1 out]
        n459 = call "Curtin_MouseBusy.vi"("VI in"=w582, "element"="LiveView", "queue in"=w581) -> ()  [unwired: 8 in, 1 out]
        n460 = property on="Device" class="Ring (strict)"("Strings []"=string[] ["Initializing..."] ("Strings [4]"), "Value"=0) -> ()  [unwired: 2 in, 2 out]
      }
      event "FRF": Shortcut Menu Activation? {
        n461 = event-data() -> ("MenuRef"=w586:refnum<k9>)  [unwired: 1 in]
        n462 = property on="Bands" class="Ring (strict)"() -> ("Value"=w583:u16)  [unwired: 2 in, 2 out]
        n463 = property on="View Type" class="Ring (strict)"() -> ("Value"=w584:u16)  [unwired: 2 in, 2 out]
        n464 = call "GenerateMenuItems.vi"("Bands"=w583, "View Type"=w584, "Menu in"=w586) -> ("error out"=w585:errorcluster)  [unwired: 8 in]
        n465 = event-data() -> ()  [unwired: 2 in, 1 out]
      }
      event "FRF": Shortcut Menu Selection (User) {
        n466 = event-data() -> ("CtlRef"=w587:refnum<vi>, "ItemTag"=w589:string)  [unwired: 1 in]
        n467 = case shown="\"savePlot\"" w589 {
          tunnel: w588 -> [_ w590 _ _ _ w600 w603 _ _ w606 w608 w610 _]
          tunnel: w587 -> [_ _ w596 w597 _ _ _ _ _ _ _ _ _]
          frame Default {
          }
          frame "toggleCentroids" {
            n468 = global read "Mic_Global.vi" "View"() -> (w594:T9)
            n469 = Unbundle By Name(w594) -> ("Centroids?"=w595:bool)
            n470 = Enqueue Element(queue=w590, element="Update") -> ()  [unwired: 2 in, 3 out]
            n471 = Not(x=w595) -> (.not. x?=w593:bool)
            n472 = Bundle By Name(cluster=w594, "Centroids?"=w593) -> (w592:T9)
            n473 = global write "Mic_Global.vi" "View"(w592) -> ()
          }
          frame "savePlot" {
            n474 = call "ExportPlots.vi"("WaveformGraph in"=w596) -> ()  [unwired: 11 in]
          }
          frame "copyImage" {
            n475 = call "GrabPlotImage.vi"("WaveformGraph in"=w597) -> ()  [unwired: 11 in]
          }
          frame "autoScale" {
            n476 = property on="dB Range" class="DigNum (strict)"() -> ("Value"=w599:dbl)  [unwired: 2 in, 2 out]
            n477 = call "AutoscaleYaxis.vi"("Has Coherence in plot?"=FALSE, "dB Range"=w599) -> ()  [unwired: 10 in]
          }
          frame "Folder" {
            n478 = Enqueue Element(queue=w600, element="Folder") -> ()  [unwired: 2 in, 3 out]
          }
          frame "saveGroup" {
            n479 = Enqueue Element(queue=w603, element="AppendAve") -> ()  [unwired: 2 in, 3 out]
          }
          frame "FontAdjust" {
            n480 = control-ref of="FRF"() -> (w604:refnum<vi>)
            n481 = call "Ask_Font.vi"("WaveformGraph in"=w604) -> ()  [unwired: 11 in]
          }
          frame "MATLAB" {
            n482 = control-ref of="FRF"() -> (w605:refnum<vi>)
            n483 = call "MATLAB.vi"("Graph"=w605) -> ()  [unwired: 10 in, 1 out]
          }
          frame "WOOD" {
            n484 = Enqueue Element(queue=w606, element="woodhouse") -> ()  [unwired: 2 in, 3 out]
          }
          frame "SAM" {
            n485 = Enqueue Element(queue=w608, element="SamZ") -> ()  [unwired: 2 in, 3 out]
          }
          frame "PLAY" {
            n486 = Enqueue Element(queue=w610, element="PlayIt") -> ()  [unwired: 2 in, 3 out]
          }
          frame "Trends" {
            n487 = control-ref of="FRF"() -> (w614:refnum<vi>)
            n488 = property on="Bands" class="Ring (strict)"() -> ("Value"=w613:u16)  [unwired: 2 in, 2 out]
            n489 = Not Equal To 0?(x=w613) -> (x != 0?=w612:bool)
            n490 = call "PlotBandsAgainstRun.vi"("Bands?"=w612, "Graph"=w614) -> ()  [unwired: 10 in]
          }
        }
      }
    }
  }
  n491 = disable-structure shown="Default" {
    disable-tunnel: [_ TRUE] -> w10
    frame condition #0 (active) {
    }
    frame condition #1 {
    }
  }
  n492 = property on="Position" class="Str"("Text.FontBold"=w10) -> ()  [unwired: 2 in, 2 out]
  n493 = disable-structure shown="RUN_TIME_ENGINE==True" {
    disable-tunnel: w9 -> [_ _]
    frame condition #0 (active) {
    }
    frame condition #1 {
      # "Stop everytng from running"
      n494 = control-ref of="This VI"() -> (w617:refnum<vi>)
      n495 = property class="VI"("FP.State"=T15."Closed" ("Front Panel Window:State")) -> (error out=w616:errorcluster)  [unwired: 2 in, 1 out]
      n496 = invoke class="VI" method="Abort VI"(reference=w617, error in=w616) -> ()  [unwired: 1 in, 3 out]
    }
  }
